vi "Actor Core.vi"(8 "error in":cluster{"状态":bool, "代码":i32, "源":string} caption="错误输入", 11 "气冷系统应用程序":refnum<class "Air Cooler Application.lvclass">) -> (0 "error out":cluster{"状态":bool, "代码":i32, "源":string} caption="错误输出", 3 "操作者输出":refnum<class "Actor.lvclass">)   [LabVIEW 2015, in "Air Cooler Application.lvlib" / "Air Cooler Application.lvclass"]
doc: "Actor Core.vi包含操作者的主要消息处理循环。操作者通常位于该循环中，在各种消息到达时对消息进行处理。如Do.vi消息返回任何错误，该循环将停止运行，错误代码43将被作为“无错误停止”的标准信号发送给调用方。如需更改上述行为，可在子孙类的Handle Error.vi中对该部分逻辑进行重写。"
uses:
  Air Cooler Application.lvclass
  <vilib>/ActorFramework/Actor/Actor.lvclass
  Cooler/Cooler/Cooler.lvclass
  Live User Controller/Live User Controller.lvclass
  <vilib>/ActorFramework/Actor/Actor.lvclass/Actor.ctl
  <vilib>/ActorFramework/Message Enqueuer/Message Enqueuer.lvclass/Message Enqueuer.ctl
  Air Cooler Application.lvclass/Air Cooler Application.ctl
  <vilib>/ActorFramework/Stop Msg/Stop Msg.lvclass/Stop Msg.ctl
  Programmatic Controller/Programmatic Controller.lvclass
  Swap Controllers Msg/Swap Controllers Msg.lvclass/Swap Controllers Msg.ctl
  Cooler Controller/Write Cooler Enqueuer Msg/Write Cooler Enqueuer Msg.lvclass/Write Cooler Enqueuer Msg.ctl
  Cooler/Write Controller Enqueuer Msg/Write Controller Enqueuer Msg.lvclass/Write Controller Enqueuer Msg.ctl
  <vilib>/ActorFramework/Message Enqueuer/Init from Existing Queue.vi
  <vilib>/ActorFramework/Message Enqueuer/Enqueue.vi
  <vilib>/ActorFramework/Message Enqueuer/Enqueue Critical.vi
  <vilib>/ActorFramework/Message Priority Queue/Priority Enqueue.vi
  <vilib>/ActorFramework/Message Enqueuer/Message Enqueuer.lvclass
  Cooler Controller/Write Cooler Enqueuer Msg/Write Cooler Enqueuer Msg.lvclass
  Cooler/Write Controller Enqueuer Msg/Write Controller Enqueuer Msg.lvclass
  <vilib>/ActorFramework/Stop Msg/Stop Msg.lvclass
  Swap Controllers Msg/Swap Controllers Msg.lvclass
panel:
  in  "DNL_Controller Selection":enum32{"UI Option 1", "UI Option 2"}(radio)
  in  "停止":bool
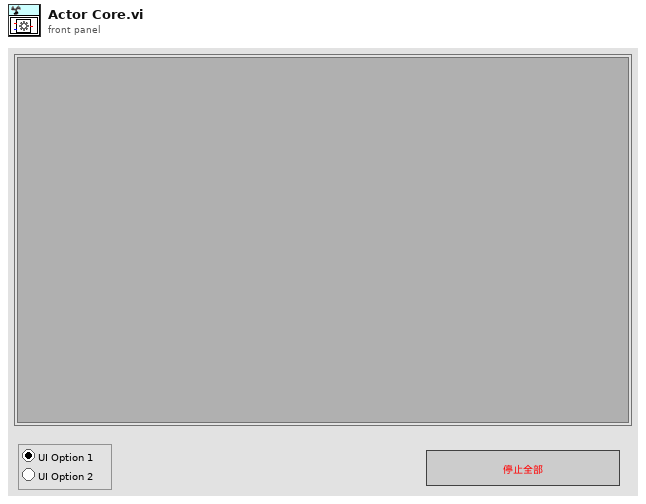
[diagram p1: front panel]
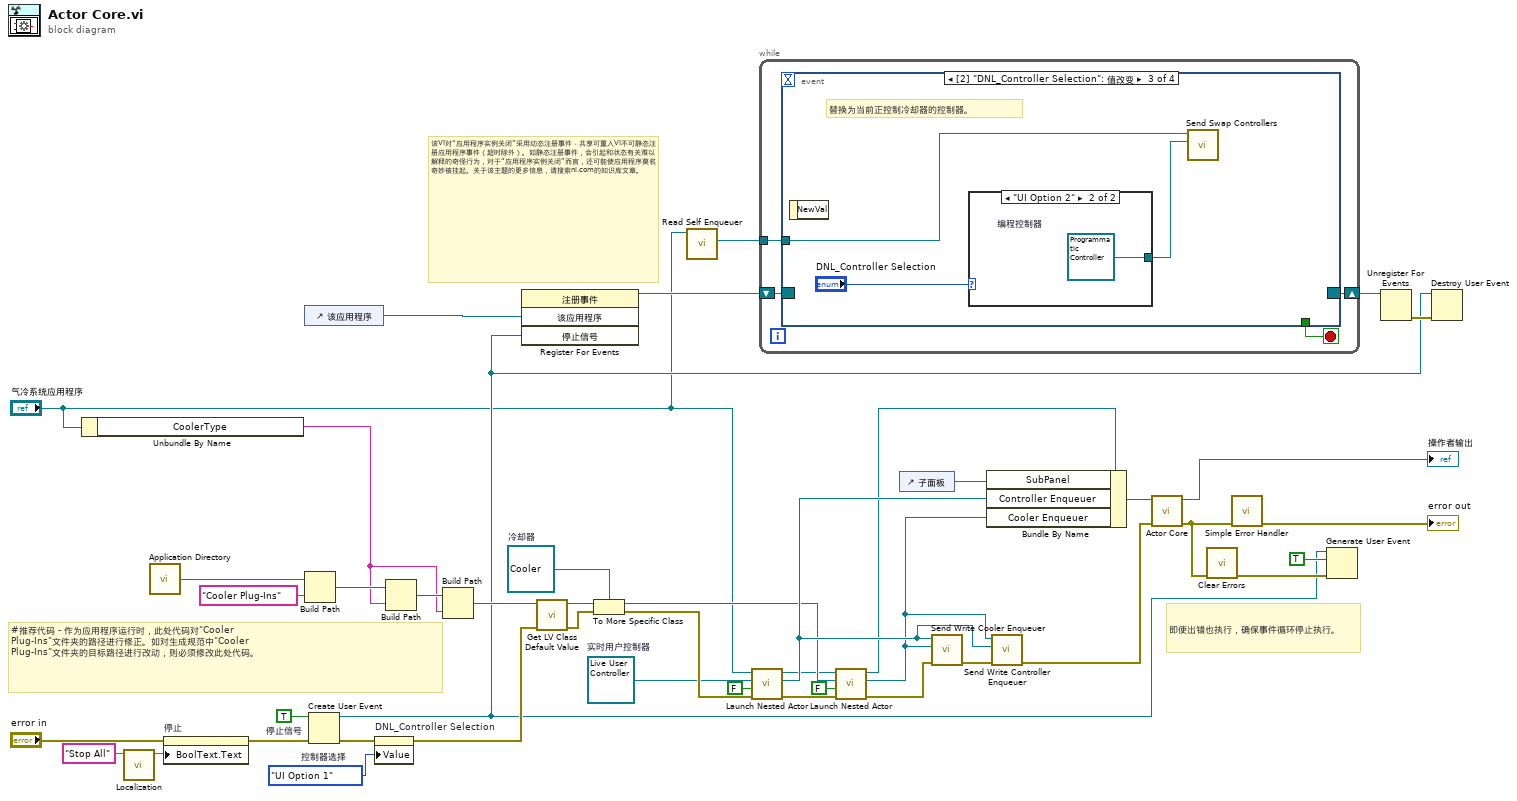
[diagram p0: block diagram]
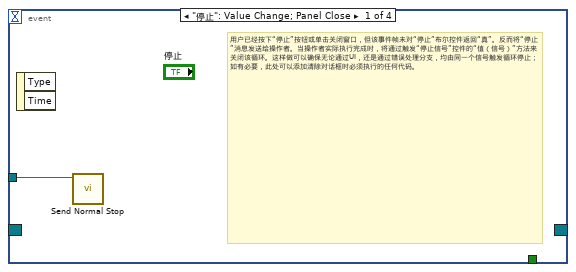
[diagram p2: hidden frame]
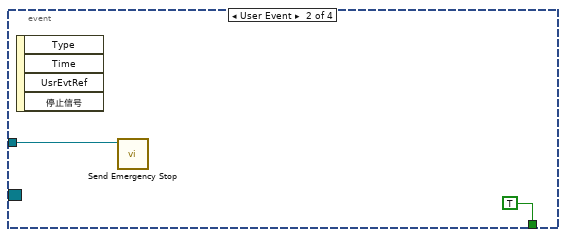
[diagram p3: hidden frame]
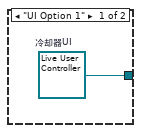
[diagram p4: hidden frame]
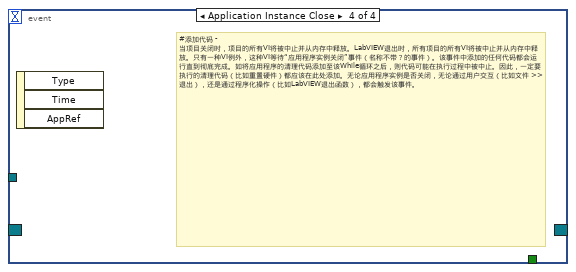
[diagram p5: hidden frame]
diagram:
  w9 = enum32{"UI Option 1", "UI Option 2"}."UI Option 1"  # 控制器选择
  w22 = TRUE  # 停止信号
  w6 = refnum<class "Live User Controller.lvclass"> refnum  # 实时用户控制器
  w34 = refnum<class "Cooler.lvclass"> refnum  # 冷却器
  # "该VI对“应用程序实例关闭”采用动态注册事件－共享可重入VI不可静态注册应用程序事件（超时除外）。如静态注册事件，会引起和状态有关难以解释的奇怪行为，对于“应用程序实例关闭”而言，还可能使应用程序莫名奇妙被挂起。关于该主题的更多信息，请搜索ni.com的知识库文章。"
  # "#推荐代码 - 作为应用程序运行时，此处代码对\"Cooler Plug-Ins\"文件夹的路径进行修正。如对生成规范中\"Cooler Plug-Ins\"文件夹的目标路径进行改动，则必须修改此处代码。"
  # "即使出错也执行，确保事件循环停止执行。"
  n1 = Unbundle By Name("气冷系统应用程序") -> ("CoolerType"=w27:string)
  n2 = call "Localization.vi"("未本地化"="Stop All" ("Unlocalized")) -> ("本地化"=w39:string)  [unwired: 10 in]
  n3 = call <vilib>:"Application Directory.vi"() -> ("Application Directory"=w10:path)
  n4 = property on="停止" class="Bool"(error in="error in", "BoolText.Text"=w39) -> (error out=w23:errorcluster)  [unwired: 1 in, 1 out]
  n5 = control-ref of="该应用程序"() -> (w11:refnum<vi>)
  n6 = Build Path(base path=w10, name or relative path="Cooler Plug-Ins") -> (appended path=w30:path)
  n7 = Create User Event(user event datatype=w22, error in=w23) -> (user event=w12:refnum<user-event>, error out=w16:errorcluster)
  n8 = property on="DNL_Controller Selection" class="RadioBtnsControl (严格)"(error in=w16, "Value"=w9) -> (error out=w15:errorcluster)  [unwired: 1 in, 1 out]
  n9 = Build Path(base path=w30, name or relative path=w27) -> (appended path=w38:path)
  n10 = Build Path(base path=w38, name or relative path=w27) -> (appended path=w37:path)
  n11 = register-events(w11, w12) -> (reference out=w21:refnum<event-registration>)  [unwired: 2 in, 1 out]
  n12 = call <vilib>:"Get LV Class Default Value.vi"("error in (no error)"=w15, "class path"=w37) -> ("error out"=w35:errorcluster, "object"=w36:refnum<class>)  [unwired: 8 in]
  n13 = To More Specific Class(target class=w34, reference=w36, error in=w35) -> (specific class reference=w8:refnum<class "Cooler.lvclass">, error out=w26:errorcluster)
  n14 = call <vilib>:"Read Self Enqueuer.vi"("Actor"="气冷系统应用程序") -> ("Self Enqueuer"=w7:refnum<class "Message Enqueuer.lvclass">)  [unwired: 10 in]
  n15 = call <vilib>:"Launch Nested Actor.vi"("error in (no error)"=w26, "Auto-stop? (T)"=FALSE, "Nested Actor"=w6, "Caller Actor in"="气冷系统应用程序") -> ("error out"=w43:errorcluster, "Nested Actor's Enqueuer"=w25:refnum<class "Message Enqueuer.lvclass">, "Caller Actor out"=w5:refnum<class "Air Cooler Application.lvclass">)  [unwired: 5 in]
  n16 = while {
    tunnel: w7 -> [w48]
    shift-right: [w45] -> w18
    shift-left: w21 -> [w46]
    stop <- w47 stop-if-true
    n17 = event shown="[2] \"DNL_Controller Selection\": 值改变" {
      selector: w46 -> [_ _ _ _]
      dyn-events: [_ _ _ _] -> w45
      timeout: _ -> [_ _ _ _]
      tunnel: w48 -> [w49 w51 w54 _]
      tunnel: [_ TRUE _ _] -> w47
      event "停止": Value Change; Panel Close {
        # "用户已经按下“停止”按钮或单击关闭窗口，但该事件帧未对“停止”布尔控件返回“真”。反而将“停止”消息发送给操作者。当操作者实际执行完成时，将通过触发“停止信号”控件的“值（信号）”方法来关闭该循环。这样做可以确保无论通过UI，还是通过错误处理分支，均由同一个信号触发循环停止；如有必要，此处可以添加清除对话框时必须执行的任何代码。"
        n18 = event-data() -> ()  [unwired: 1 in, 2 out]
        n19 = call <vilib>:"Send Normal Stop.vi"("Message Enqueuer"=w49) -> ()  [unwired: 10 in, 1 out]
      }
      event User Event {
        n20 = event-data() -> ()  [unwired: 1 in, 4 out]
        n21 = call <vilib>:"Send Emergency Stop.vi"("Message Enqueuer"=w51) -> ()  [unwired: 10 in, 1 out]
      }
      event "DNL_Controller Selection": Value Change {
        # "替换为当前正控制冷却器的控制器。"
        n22 = event-data() -> ()  [unwired: 1 in, 1 out]
        n23 = case shown="\"UI Option 2\"" "DNL_Controller Selection" {
          tunnel: [w55 w56] -> w52
          frame "UI Option 1" {
            w55 = refnum<class "Live User Controller.lvclass"> refnum  # 冷却器UI
          }
          frame "UI Option 2" {
            w56 = refnum<class "Programmatic Controller.lvclass"> refnum  # 编程控制器
          }
        }
        n24 = call "Send Swap Controllers.vi"("冷却器控制器"=w52, "消息待入队列"=w54) -> ()  [unwired: 9 in, 1 out]
      }
      event Application Instance Close {
        # "#添加代码 - 当项目关闭时，项目的所有VI将被中止并从内存中释放。LabVIEW退出时，所有项目的所有VI将被中止并从内存中释放。只有一种VI例外，这种VI等待“应用程序实例关闭”事件（名称不带？的事件）。该事件中添加的任何代码都会运行直到彻底完成。如将应用程序的清理代码添加至该While循环之后，则代码可能在执行过程中被中止。因此，一定要执行的清理代码（比如重置硬件）都应该在此处添加。无论应用程序实例是否关闭，无论通过用户交互（比如文件 >> 退出），还是通过程序化操作（比如LabVIEW退出函数），都会触发该事件。"
        n25 = event-data() -> ()  [unwired: 1 in, 3 out]
      }
    }
  }
  n26 = call <vilib>:"Launch Nested Actor.vi"("error in (no error)"=w43, "Auto-stop? (T)"=FALSE, "Nested Actor"=w8, "Caller Actor in"=w5) -> ("error out"=w32:errorcluster, "Nested Actor's Enqueuer"=w24:refnum<class "Message Enqueuer.lvclass">, "Caller Actor out"=w3:refnum<class "Air Cooler Application.lvclass">)  [unwired: 5 in]
  n27 = control-ref of="子面板"() -> (w33:refnum<vi>)
  n28 = call "Send Write Cooler Enqueuer.vi"("error in (no error)"=w32, "冷却器待入队列"=w24, "消息待入队列"=w25) -> ("error out"=w29:cluster{"状态":bool, "代码":i32, "源":string})  [unwired: 8 in]
  n29 = Bundle By Name(cluster=w3, "SubPanel"=w33, "Controller Enqueuer"=w25, "Cooler Enqueuer"=w24) -> (w42:refnum<class "Air Cooler Application.lvclass">)
  n30 = call "Send Write Controller Enqueuer.vi"("error in (no error)"=w29, "控制器待入队列"=w25, "消息待入队列"=w24) -> ("error out"=w28:cluster{"状态":bool, "代码":i32, "源":string})  [unwired: 8 in]
  n31 = call-parent "Actor Core.vi"("error in"=w28, "Actor in"=w42) -> ("error out"=w14:errorcluster, "Actor out"=→"操作者输出":refnum<class "Actor.lvclass">)  [unwired: 8 in]
  n32 = call <vilib>:"Clear Errors.vi"("error in (no error)"=w14) -> ("error out"=w20:errorcluster)  [unwired: 5 in, 1 out]
  n33 = call <vilib>:"Simple Error Handler.vi"("error in (no error)"=w14) -> ("error out"=→"error out":errorcluster)  [unwired: 4 in, 4 out]
  n34 = Generate User Event(user event=w12, event data cluster=TRUE ("stop"), error in=w20) -> ()  [unwired: 1 in, 2 out]
  n35 = Unregister For Events(event registration refnum=w18) -> (error out=w17:errorcluster)  [unwired: 1 in]
  n36 = Destroy User Event(user event=w12, error in=w17) -> ()  [unwired: 1 out]
